vi "Get Sender.vi"(8 "error in (no error)":errorcluster, 11 "Message in":refnum<class "Message.lvclass">) -> (0 "error out":errorcluster, 2 "Sender":refnum<class "Endpoint.lvclass">, 3 "Message out":refnum<class "Message.lvclass">)   [LabVIEW 2020, in "Stream-Simple-Msg.lvlib" / "Message.lvclass"]
doc: "Provides the Enpoint instance that represents the sender of the message. This can be useful to get more information about the sender such as the URI string identifying the sender and send replies to the sender. For replying, a convenience Message:Reply VI exists to simplify the interaction."
uses:
  Message.lvclass
  Endpoint/Endpoint.lvclass
  Message.lvclass/Message.ctl
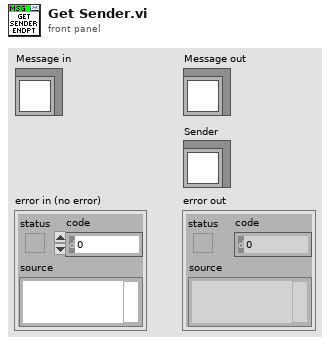
[diagram p1: front panel]
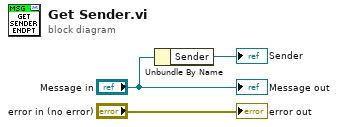
[diagram p0: block diagram]
diagram:
  n1 = Unbundle By Name("Message in") -> ("Sender"=→"Sender":refnum<class "Endpoint.lvclass">)
  "error out" <- "error in (no error)"
  "Message out" <- "Message in"
